vi "Senzor_ploaie.vi"() -> ()   [LabVIEW 2018]
uses:
  <vilib>/MakerHub/LINX/Public/Peripherals/Analog/Analog Read 1 Chan.vi
  <vilib>/MakerHub/LINX/Public/Peripherals/Analog/Analog Read N Chans.vi
  <vilib>/MakerHub/LINX/Private/Local IO/LinxAnalogRead.vi
  <vilib>/MakerHub/LINX/Public/Utilities/Check Channel.vi
  <vilib>/Utility/file.llb/Write Delimited Spreadsheet (string).vi
  <vilib>/MakerHub/LINX/Public/Utilities/Open Serial.vi
  <vilib>/Utility/file.llb/Write Delimited Spreadsheet (DBL).vi
  <vilib>/MakerHub/LINX/Private/Utilties/Generate Error.vi
  <vilib>/MakerHub/LINX/LMH-LINX.lvlib
panel:
  in  "?":bool
  in  "Serial Port":refnum<visa-resource-name>="N/A"
  out "file or folder exists?":bool
  out "AI Ref":dbl
  out "Voltage":dbl
  out "Senzor\nploaie":dbl caption="x*y 2"
  out "date/time string":string
  out "Senzor ploaie 2":dbl(graph)
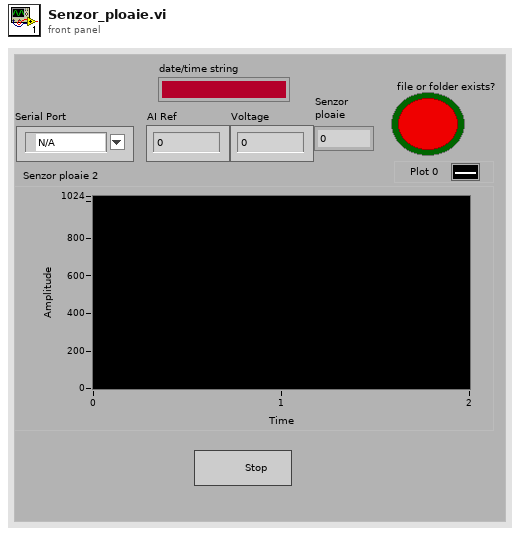
[diagram p1: front panel]
types:
  T1 = enum16{"open", "replace", "create", "open or create", "replace or create", "replace or create with confirmation"}
  T2 = typedef "LMH-LINX.lvlib/LINX Ref.ctl" = cluster{"IO":T3, "Interface":T4, "LINX Device Config":T5}
  T3 = typedef "LMH-LINX.lvlib/Platform.ctl" = enum16{"Remote", "Local"}
  T4 = typedef "LMH-LINX.lvlib/Interface.ctl" = enum16{"Serial", "TCP"}
  T5 = typedef "LMH-LINX.lvlib/Device.lvlib/LINX Device Config.ctl" = cluster{"Interface":T4, "COM Port":refnum<visa-resource-name>, "TCP Configuration":T6, "Device Family":u8, "Device ID":u8, "Device Name":string, "TCP Ref":refnum<k5>, "Channels":T7}
  T6 = typedef "LMH-LINX.lvlib/Device.lvlib/TCP Config.ctl" = cluster{"IP Address":string, "Port":u16}
  T7 = typedef "LMH-LINX.lvlib/Channels.ctl" = cluster{"DI":u8[], "DO":u8[], "AI":u8[], "AO":u8[], "PWM":u8[], "QE":u8[], "UART":u8[], "I2C 2":u8[], "SPI":u8[], "CAN":u8[], "Servo":u8[], "AI Ref (V)":dbl, "AI Resolution (Bits)":u8, "AO Ref (V)":dbl, "AO Resolution (Bits)":u8}
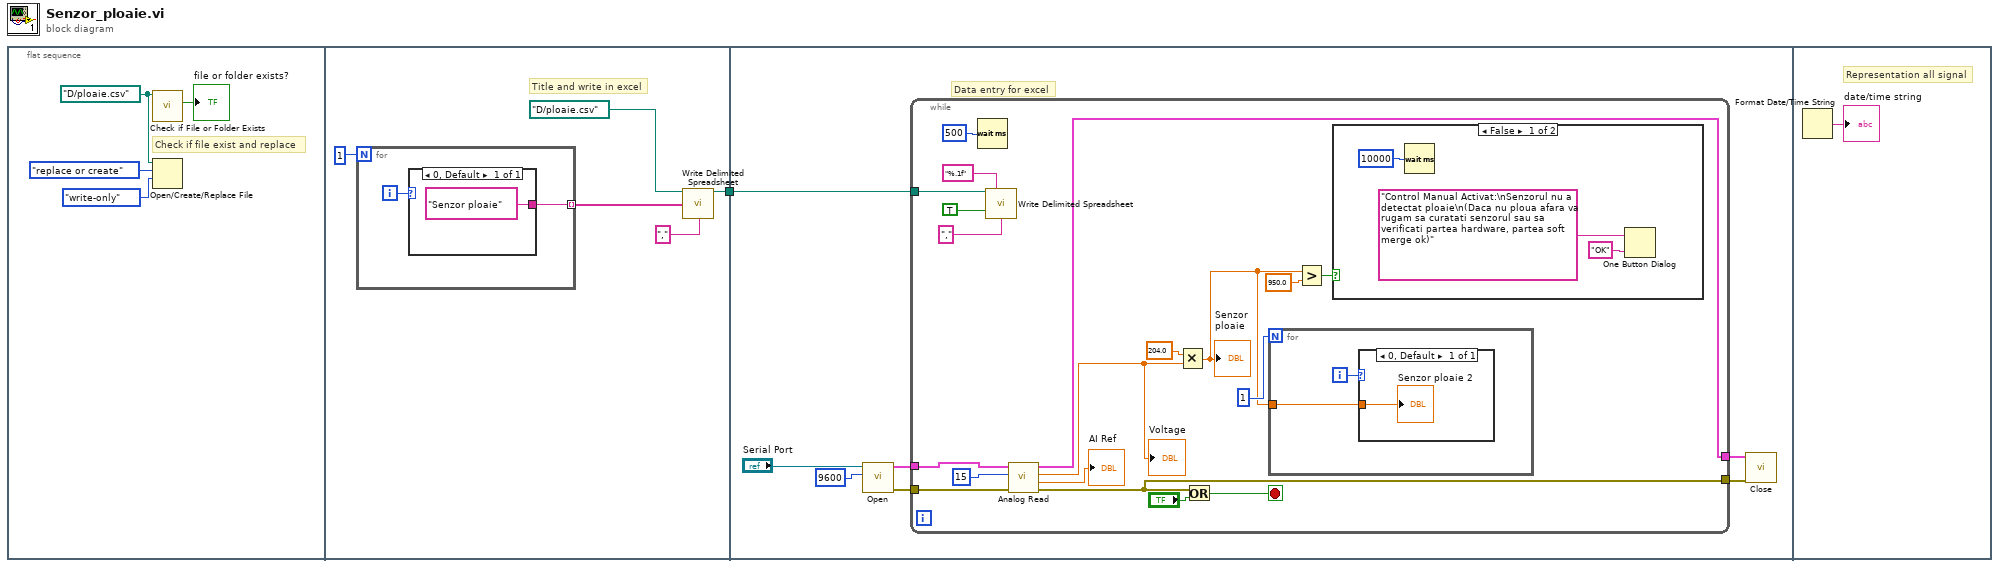
[diagram p0: block diagram]
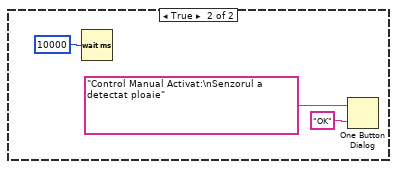
[diagram p2: hidden frame]
diagram:
  n1 = flat-sequence {
    tunnel: [w9] -> w1
    tunnel: w1 -> [w14]
    frame #0 {
      w4 = path "D:/ploaie.csv" ("path")
      # "Check if file exist and replace"
      n2 = call <vilib>:"Check if File or Folder Exists.vi"("path"=w4) -> ("file or folder exists?"=→"file or folder exists?":bool)  [unwired: 8 in, 2 out]
      n3 = Open/Create/Replace File(file path (use dialog)=w4, operation (0:open)=T1."replace or create", access (0:read/write)=enum16{"read/write", "read-only", "write-only"}."write-only") -> ()  [unwired: 3 in, 3 out]
    }
    frame #1 {
      # "Title and write in excel"
      n4 = for {
        N: 1 -> [_]
        tunnel: [w11] -> w6 mode=indexing
        i -> [w12]
        n5 = case shown="0, Default" w12 {
          tunnel: ["Senzor ploaie"] -> w11
          frame 0, Default {
          }
        }
      }
      n6 = call-poly <vilib>:"Write Delimited Spreadsheet.vi"("file path (dialog if empty)"=path "D:/ploaie.csv", "1D data"=w6, "delimiter (\\t)"="," ("delimiter (\\t)")) -> ("new file path (Not A Path if cancelled)"=w9:path)  [unwired: 11 in, 1 out]
    }
    frame #2 {
      # "Data entry for excel"
      n7 = call-poly <vilib>:"Open.vi"("Baud Rate Override"=u32 9600, "Serial Port"="Serial Port") -> ("Error Out"=w19:errorcluster, "LINX Resource"=w20:T2)  [unwired: 7 in, 1 out]
      n8 = while {
        tunnel: w20 -> [w36]
        tunnel: w19 -> [w35]
        tunnel: [w34] -> w18
        tunnel: [w33] -> w17
        tunnel: w14 -> [w24]
        stop <- w39 stop-if-true
        n9 = Wait (ms)(milliseconds to wait=u32 500) -> ()  [unwired: 1 out]
        n10 = call-poly <vilib>:"Write Delimited Spreadsheet.vi"("file path (dialog if empty)"=w24, "format (%.3f)"="%.1f", "append to file? (new file:F)"=TRUE, "delimiter (\\t)"="," ("delimiter (\\t)")) -> ()  [unwired: 10 in, 2 out]
        n11 = call-poly <vilib>:"Analog Read.vi"("Error In"=w35, "Analog Channel"=u8 15, "LINX Resource"=w36) -> ("Error Out"=w33:errorcluster, "AI Ref"=→"AI Ref":dbl, "Voltage"=w30:dbl, "LINX Resource"=w34:T2)  [unwired: 5 in]
        "Voltage" <- w30
        n12 = Multiply(x=204.0, y=w30) -> (x*y=w25:dbl)
        "Senzor\nploaie" <- w25
        n13 = Or(x=w33, y="?") -> (x .or. y?=w39:bool)
        n14 = for {
          N: 1 -> [_]
          tunnel: w25 -> [w40]
          i -> [w41]
          n15 = case shown="0, Default" w41 {
            tunnel: w40 -> [w42]
            frame 0, Default {
              "Senzor ploaie 2" <- w42
            }
          }
        }
        n16 = Greater?(x=w25, y=950.0) -> (0:w28:bool)
        n17 = case shown="False" w28 {
          frame False {
            n18 = Wait (ms)(milliseconds to wait=u32 10000) -> ()  [unwired: 1 out]
            n19 = One Button Dialog(message="Control Manual Activat:\nSenzorul nu a detectat ploaie\n(Daca nu ploua afara va rugam sa curatati senzorul sau sa verificati partea hardware, partea soft merge ok)", button name ("OK")="OK") -> ()  [unwired: 1 out]
          }
          frame True {
            n20 = Wait (ms)(milliseconds to wait=u32 10000) -> ()  [unwired: 1 out]
            n21 = One Button Dialog(message="Control Manual Activat:\nSenzorul a detectat ploaie", button name ("OK")="OK") -> ()  [unwired: 1 out]
          }
        }
      }
      n22 = call <vilib>:"Close.vi"("Error In"=w17, "LINX Resource"=w18) -> ()  [unwired: 9 in, 1 out]
    }
    frame #3 {
      # "Representation all signal"
      n23 = Format Date/Time String() -> (date/time string=→"date/time string":string)  [unwired: 3 in]
    }
  }
